vi "ReversedEngineering GetDiagramSubVIs.vi"(0 "Diagram":refnum<vi>, 1 "SubVIsOptions(NormalSubVis)":T1(ring), 2 "RecrsiveSearchInNormalSubVIs(False)":bool, 5 "error in (no error)":errorcluster, 9 "PathToDebugVI(OnlyUsedForRecursivVitFiles)":path) -> (14 "DiagramOut":refnum<vi>, 15 "SubViNames":string[](array[string]), 19 "error out":errorcluster)   [LabVIEW 2020]
panel:
  in  "Debug?":bool
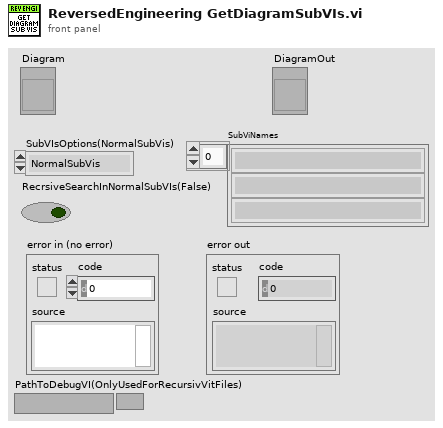
[diagram p1: front panel]
types:
  T1 = enum16{"NormalSubVis", "LV-Internal VIs", "All VIs", "All Functions"}
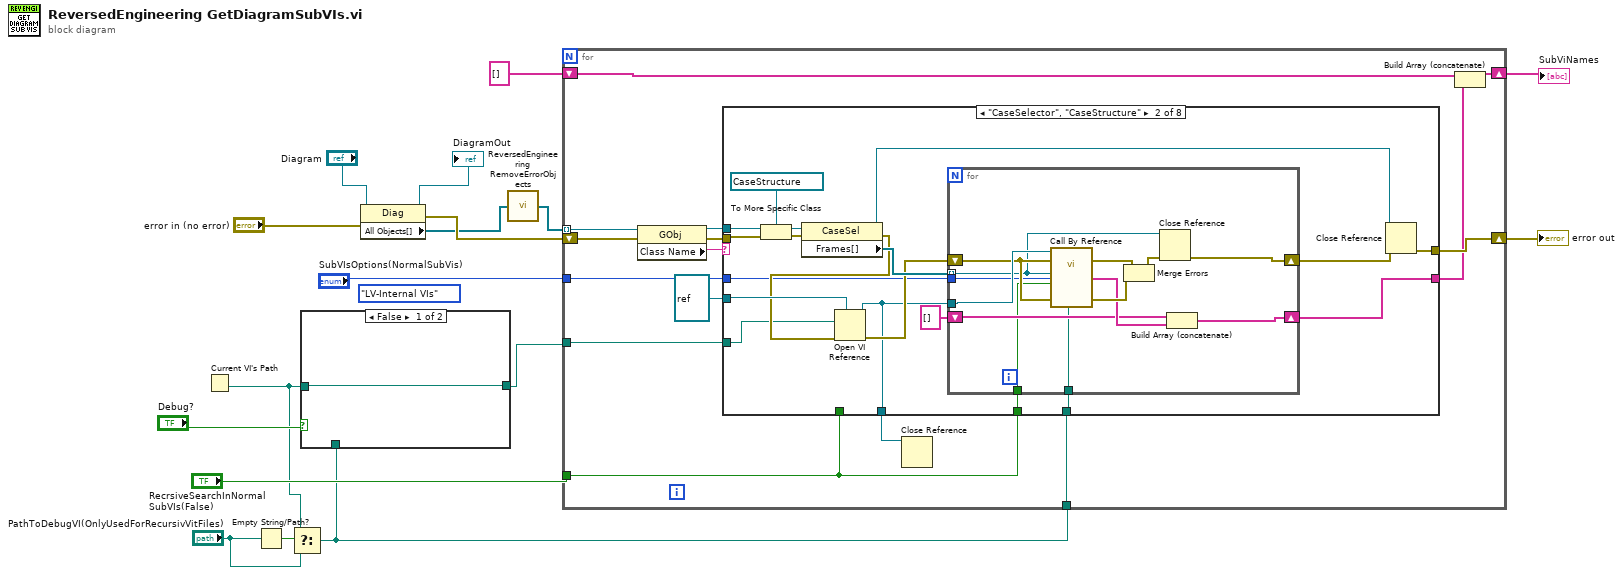
[diagram p0: block diagram]
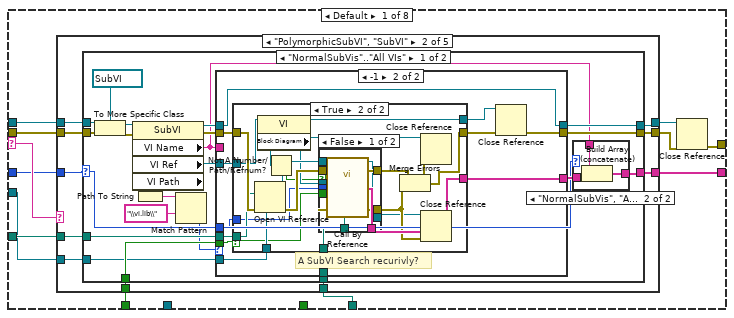
[diagram p2: hidden frame]
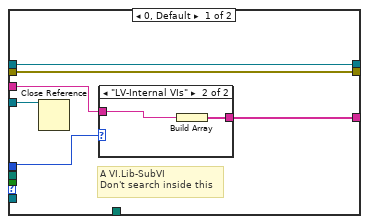
[diagram p5: hidden frame]
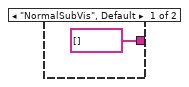
[diagram p6: hidden frame]
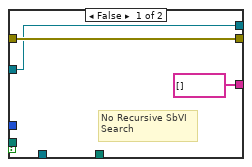
[diagram p7: hidden frame]
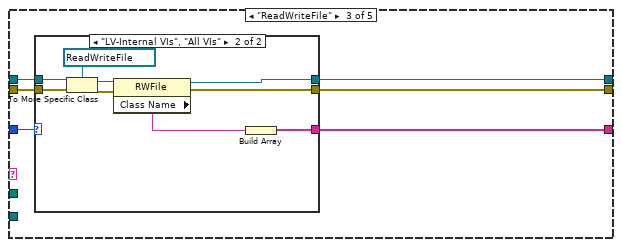
[diagram p10: hidden frame]
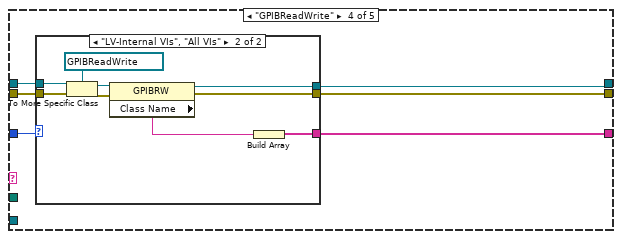
[diagram p12: hidden frame]
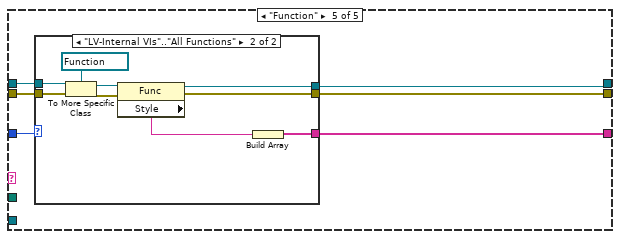
[diagram p14: hidden frame]
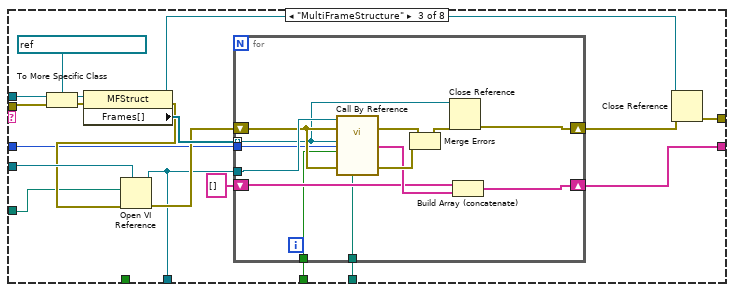
[diagram p16: hidden frame]
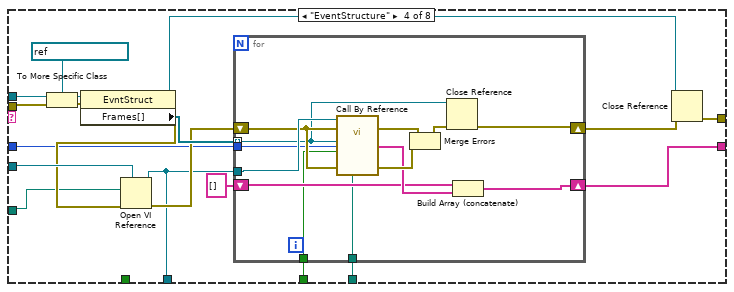
[diagram p17: hidden frame]
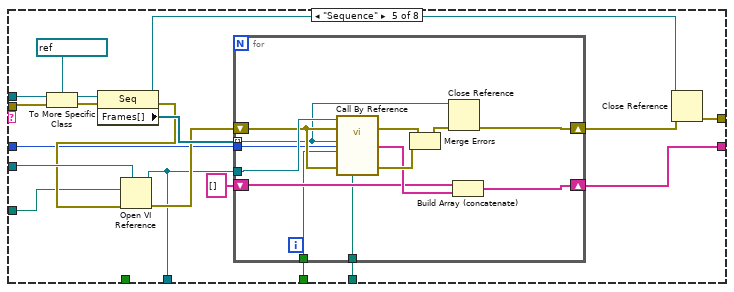
[diagram p18: hidden frame]
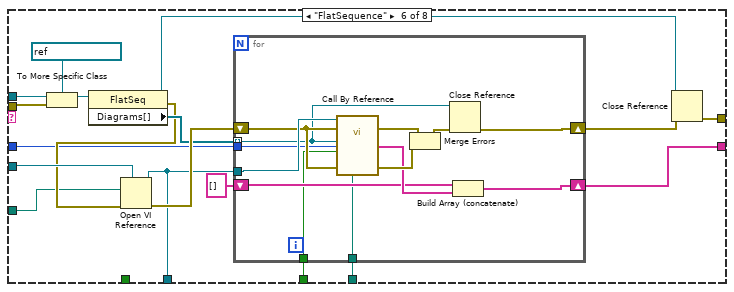
[diagram p19: hidden frame]
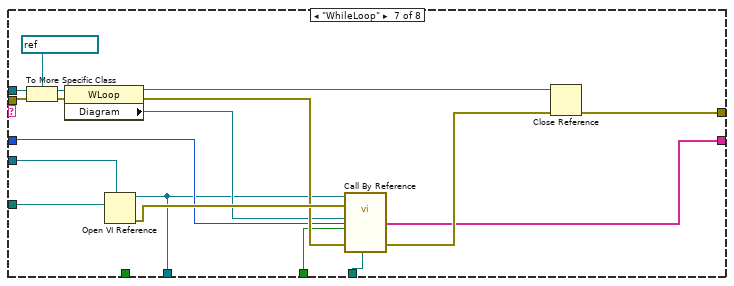
[diagram p20: hidden frame]
diagram:
  (unwired) T1."LV-Internal VIs" ("SubVIsOptions(NormalSubVis)")
  n1 = Current VI's Path() -> (path=w5:path)
  n2 = Empty String/Path?(string/path="PathToDebugVI(OnlyUsedForRecursivVitFiles)") -> (empty?=w6:bool)
  n3 = Select(t=w5, s=w6, f="PathToDebugVI(OnlyUsedForRecursivVitFiles)") -> (s? t:f=w3:path)
  n4 = case shown="False" "Debug?" {
    tunnel: w5 -> [w18 _]
    tunnel: [w18 w24] -> w8
    tunnel: w3 -> [_ w21]
    frame False {
    }
    frame True {
      n5 = Strip Path(path=w21) -> (stripped path=w19:path, name=w20:string)
      n6 = Concatenate Strings(w20, "t" ("f")) -> (w23:string)
      n7 = Build Path(base path=w19, name or relative path=w23) -> (appended path=w24:path)
    }
  }
  n8 = property class="Diag"(reference="Diagram", error in="error in (no error)") -> (reference out=→"DiagramOut":refnum<vi>, error out=w15:errorcluster, "All Objects[]"=w2:refnum<vi>[])
  n9 = call <resource>:"ReversedEngineering RemoveErrorObjects.vi"("ObjectsIn"=w2) -> ("ObjectsOut"=w1:refnum<vi>[])
  n10 = for {
    tunnel: w1 -> [w25] mode=indexing
    shift-right: [w38] -> w14
    shift-left: w15 -> [w39]
    shift-right: [w37] -> w13
    shift-left: string[] [] -> [w31]
    tunnel: w8 -> [w35]
    tunnel: "SubVIsOptions(NormalSubVis)" -> [w34]
    tunnel: "RecrsiveSearchInNormalSubVIs(False)" -> [w33]
    tunnel: w3 -> [w32]
    n11 = property class="GObj"(reference=w25, error in=w39) -> (reference out=w29:refnum<vi>, error out=w28:errorcluster, "Class Name"=w30:string)
    n12 = case shown="\"CaseSelector\", \"CaseStructure\"" w30 {
      selector: w30 -> [w50 _ _ _ _ _ _ _]
      tunnel: w29 -> [w48 w214 w246 w278 w310 w341 w372 w390]
      tunnel: w28 -> [w49 w209 w242 w274 w306 w340 w366 w384]
      tunnel: [w51 w208 w241 w273 w305 w339 w356 w374] -> w38
      tunnel: [w45 w202 w235 w267 w300 w335 w362 w380] -> w36
      tunnel: refnum<vi> refnum ("VI Refnum") -> [w41 w205 w238 w270 w302 w337 w361 w379]
      tunnel: w35 -> [w42 w200 w232 w264 w297 w328 w360 w378]
      tunnel: [_ w199 w231 w263 w295 w327 w355 w373] -> w26
      tunnel: w34 -> [w44 w198 w230 w262 w294 w326 w359 w377]
      tunnel: w33 -> [_ w197 w229 w261 w293 w325 w358 w376]
      tunnel: w33 -> [w43 _ _ _ _ _ _ _]
      tunnel: w32 -> [w40 w196 w228 w260 w292 w324 w357 w375]
      frame Default {
        n13 = case shown="\"PolymorphicSubVI\", \"SubVI\"" w50 {
          tunnel: w49 -> [w53 w62 w149 w166 w183]
          tunnel: w48 -> [w52 w63 w150 w167 w184]
          tunnel: [w53 w60 w147 w162 w179] -> w47
          tunnel: [w52 w59 w146 w164 w181] -> w46
          tunnel: [_ w61 w148 w165 w182] -> w45
          tunnel: w44 -> [_ w58 w145 w163 w180]
          tunnel: w43 -> [_ w57 _ _ _]
          tunnel: w42 -> [_ w56 _ _ _]
          tunnel: w41 -> [_ w55 _ _ _]
          tunnel: w40 -> [_ w54 _ _ _]
          frame "False", Default {
          }
          frame "PolymorphicSubVI", "SubVI" {
            n14 = case shown="\"NormalSubVis\"..\"All VIs\"" w58 {
              selector: w58 -> [w66 _]
              tunnel: w63 -> [w84 w144]
              tunnel: w62 -> [w83 w143]
              tunnel: [w81 _] -> w61
              tunnel: [w73 w143] -> w60
              tunnel: [w74 w144] -> w59
              tunnel: w57 -> [w71 _]
              tunnel: w56 -> [w70 _]
              tunnel: w55 -> [w68 _]
              tunnel: w54 -> [w67 _]
              frame "NormalSubVis".."All VIs" {
                n15 = To More Specific Class(target class=refnum<vi> refnum ("WhileLoop"), reference=w84, error in=w83) -> (specific class reference=w82:refnum<vi>, error out=w80:errorcluster)
                n16 = property class="SubVI"(reference=w82, error in=w80) -> (reference out=w75:refnum<vi>, error out=w76:errorcluster, "VI Name"=w64:string, "VI Ref"=w69:refnum<vi>, "VI Path"=w79:path)
                n17 = Path To String(path=w79) -> (string=w78:string)
                n18 = Match Pattern(string=w78, regular expression="\\vi.lib\\") -> (offset past match=w65:i32)  [unwired: 4 out]
                n19 = case shown="-1" w65 {
                  tunnel: w76 -> [w94 w109]
                  tunnel: w75 -> [w95 w102]
                  tunnel: [w95 w102] -> w74
                  tunnel: [w94 w100] -> w73
                  tunnel: [w92 w108] -> w72
                  tunnel: w71 -> [_ w110]
                  tunnel: w70 -> [_ w107]
                  tunnel: w69 -> [w93 w106]
                  tunnel: w68 -> [_ w105]
                  tunnel: w67 -> [_ w104]
                  tunnel: w66 -> [w91 w103]
                  tunnel: w64 -> [w90 _]
                  frame 0, Default {
                    # "A VI.Lib-SubVI\nDon't search inside this"
                    n20 = Close Reference(reference=w93) -> ()  [unwired: 1 in, 1 out]
                    n21 = case shown="\"LV-Internal VIs\"" w91 {
                      tunnel: [string[] [] w98] -> w92
                      tunnel: w90 -> [_ w97]
                      frame "NormalSubVis", Default {
                      }
                      frame "LV-Internal VIs" {
                        n22 = Build Array(w97) -> (w98:string[])
                      }
                    }
                  }
                  frame -1 {
                    # "A SubVI Search recurivly?"
                    n23 = case shown="True" w110 {
                      selector: w110 -> [_ w121]
                      tunnel: w109 -> [w113 w128]
                      tunnel: [w113 w115] -> w101
                      tunnel: [string[] [] ("appended array") w123] -> w108
                      tunnel: w107 -> [_ w127]
                      tunnel: w106 -> [w111 w125]
                      tunnel: w105 -> [_ w124]
                      tunnel: w103 -> [_ w122]
                      tunnel: w104 -> [_ w118]
                      tunnel: [w111 w114] -> w99
                      frame False {
                        # "No Recursive SbVI\nSearch"
                      }
                      frame True {
                        n24 = Open VI Reference(type specifier VI Refnum (for type only)=w124, vi path=w127, error in (no error)=w128) -> (vi reference=w126:refnum<vi>, error out=w129:errorcluster)  [unwired: 3 out]
                        n25 = property class="VI"(reference=w125) -> (reference out=w114:refnum<vi>, "Block Diagram"=w117:refnum<vi>)  [unwired: 1 in, 1 out]
                        n26 = Not A Number/Path/Refnum?(number/path/refnum=w117) -> (NaN/Path/Refnum?=w116:bool)
                        n27 = case shown="False" w116 {
                          tunnel: [w140 w142] -> w130
                          tunnel: w129 -> [w139 w142]
                          tunnel: w126 -> [w138 w141]
                          tunnel: w117 -> [w137 _]
                          tunnel: [w136 _] -> w123
                          tunnel: w122 -> [w135 _]
                          tunnel: w121 -> [w134 _]
                          tunnel: [w133 _] -> w120
                          tunnel: [w132 w141] -> w119
                          tunnel: w118 -> [w131 _]
                          frame False {
                            n28 = call-by-ref "?"(reference=w138, error in=w139, "Diagram"=w137, "SubVIsOptions(NormalSubVis)"=w135, "RecrsiveSearchInNormalSubVIs(False)"=w134, "error in (no error)"=w139, "PathToDebugVI(OnlyUsedForRecursivVitFiles)"=w131) -> (reference out=w132:refnum<vi>, error out=w140:errorcluster, "SubViNames"=w136:string[], 19:"error out"=w133:errorcluster)  [unwired: 12 in, 1 out]
                          }
                          frame True {
                          }
                        }
                        n29 = Merge Errors(w130, w120) -> (w115:errorcluster)
                        n30 = Close Reference(reference=w117, error in (no error)=w115) -> ()  [unwired: 1 out]
                        n31 = Close Reference(reference=w119, error in (no error)=w120) -> ()  [unwired: 1 out]
                      }
                    }
                    n32 = Close Reference(reference=w99, error in (no error)=w101) -> (error out=w100:errorcluster)
                  }
                }
                n33 = case shown="\"NormalSubVis\", \"All VIs\"" w66 {
                  tunnel: [w86 w89] -> w81
                  tunnel: w64 -> [_ w88]
                  tunnel: w72 -> [w86 w87]
                  frame Default {
                  }
                  frame "NormalSubVis", "All VIs" {
                    n34 = Build Array (concatenate)(w88, w87) -> (w89:string[])
                  }
                }
              }
              frame Default {
              }
            }
          }
          frame "ReadWriteFile" {
            n35 = case shown="\"LV-Internal VIs\", \"All VIs\"" w145 {
              tunnel: w150 -> [w152 w160]
              tunnel: w149 -> [w151 w159]
              tunnel: [_ w156] -> w148
              tunnel: [w151 w155] -> w147
              tunnel: [w152 w154] -> w146
              frame Default {
              }
              frame "LV-Internal VIs", "All VIs" {
                n36 = To More Specific Class(target class=refnum<vi> refnum ("WhileLoop"), reference=w160, error in=w159) -> (specific class reference=w158:refnum<vi>, error out=w153:errorcluster)
                n37 = property class="RWFile"(reference=w158, error in=w153) -> (reference out=w154:refnum<vi>, error out=w155:errorcluster, "Class Name"=w157:string)
                n38 = Build Array(w157) -> (w156:string[])
              }
            }
          }
          frame "GPIBReadWrite" {
            n39 = case shown="\"LV-Internal VIs\", \"All VIs\"" w163 {
              tunnel: w167 -> [w169 w177]
              tunnel: w166 -> [w168 w176]
              tunnel: [_ w173] -> w165
              tunnel: [w169 w172] -> w164
              tunnel: [w168 w170] -> w162
              frame Default {
              }
              frame "LV-Internal VIs", "All VIs" {
                n40 = To More Specific Class(target class=refnum<vi> refnum ("WhileLoop"), reference=w177, error in=w176) -> (specific class reference=w175:refnum<vi>, error out=w171:errorcluster)
                n41 = property class="GPIBRW"(reference=w175, error in=w171) -> (reference out=w172:refnum<vi>, error out=w170:errorcluster, "Class Name"=w174:string)
                n42 = Build Array(w174) -> (w173:string[])
              }
            }
          }
          frame "Function" {
            n43 = case shown="\"LV-Internal VIs\"..\"All Functions\"" w180 {
              tunnel: w184 -> [w186 w194]
              tunnel: w183 -> [w185 w193]
              tunnel: [_ w190] -> w182
              tunnel: [w186 w189] -> w181
              tunnel: [w185 w187] -> w179
              frame Default {
              }
              frame "LV-Internal VIs".."All Functions" {
                n44 = To More Specific Class(target class=refnum<vi> refnum ("WhileLoop"), reference=w194, error in=w193) -> (specific class reference=w192:refnum<vi>, error out=w188:errorcluster)
                n45 = property class="Func"(reference=w192, error in=w188) -> (reference out=w189:refnum<vi>, error out=w187:errorcluster, "Style"=w191:string)
                n46 = Build Array(w191) -> (w190:string[])
              }
            }
          }
        }
        n47 = Close Reference(reference=w46, error in (no error)=w47) -> (error out=w51:errorcluster)
      }
      frame "CaseSelector", "CaseStructure" {
        n48 = To More Specific Class(target class=refnum<vi> refnum ("CaseSelector"), reference=w214, error in=w209) -> (specific class reference=w212:refnum<vi>, error out=w210:errorcluster)
        n49 = property class="CaseSel"(reference=w212, error in=w210) -> (reference out=w206:refnum<vi>, error out=w204:errorcluster, "Frames[]"=w211:refnum<vi>[])
        n50 = Open VI Reference(type specifier VI Refnum (for type only)=w205, vi path=w200, error in (no error)=w204) -> (vi reference=w199:refnum<vi>, error out=w207:errorcluster)  [unwired: 3 out]
        n51 = for {
          tunnel: w211 -> [w218] mode=indexing
          shift-right: [w220] -> w203
          shift-left: w207 -> [w225]
          tunnel: w199 -> [w226]
          shift-right: [w221] -> w202
          shift-left: string[] [] -> [w222]
          tunnel: w198 -> [w217]
          tunnel: w197 -> [w216]
          tunnel: w196 -> [w215]
          n52 = call-by-ref "?"(reference=w226, error in=w225, "Diagram"=w218, "SubVIsOptions(NormalSubVis)"=w217, "RecrsiveSearchInNormalSubVIs(False)"=w216, "error in (no error)"=w225, "PathToDebugVI(OnlyUsedForRecursivVitFiles)"=w215) -> (error out=w227:errorcluster, "SubViNames"=w223:string[], 19:"error out"=w224:errorcluster)  [unwired: 12 in, 2 out]
          n53 = Merge Errors(w227, w224) -> (w219:errorcluster)
          n54 = Close Reference(reference=w218, error in (no error)=w219) -> (error out=w220:errorcluster)
          n55 = Build Array (concatenate)(w222, w223) -> (w221:string[])
        }
        n56 = Close Reference(reference=w206, error in (no error)=w203) -> (error out=w208:errorcluster)
      }
      frame "MultiFrameStructure" {
        n57 = To More Specific Class(target class=refnum<vi> refnum ("MultiFrameStructure"), reference=w246, error in=w242) -> (specific class reference=w245:refnum<vi>, error out=w243:errorcluster)
        n58 = property class="MFStruct"(reference=w245, error in=w243) -> (reference out=w239:refnum<vi>, error out=w237:errorcluster, "Frames[]"=w244:refnum<vi>[])
        n59 = Open VI Reference(type specifier VI Refnum (for type only)=w238, vi path=w232, error in (no error)=w237) -> (vi reference=w231:refnum<vi>, error out=w240:errorcluster)  [unwired: 3 out]
        n60 = for {
          tunnel: w244 -> [w252] mode=indexing
          shift-right: [w250] -> w236
          shift-left: w240 -> [w257]
          tunnel: w231 -> [w258]
          shift-right: [w253] -> w235
          shift-left: string[] [] -> [w254]
          tunnel: w230 -> [w249]
          tunnel: w229 -> [w248]
          tunnel: w228 -> [w247]
          n61 = call-by-ref "?"(reference=w258, error in=w257, "Diagram"=w252, "SubVIsOptions(NormalSubVis)"=w249, "RecrsiveSearchInNormalSubVIs(False)"=w248, "error in (no error)"=w257, "PathToDebugVI(OnlyUsedForRecursivVitFiles)"=w247) -> (error out=w259:errorcluster, "SubViNames"=w255:string[], 19:"error out"=w256:errorcluster)  [unwired: 12 in, 2 out]
          n62 = Merge Errors(w259, w256) -> (w251:errorcluster)
          n63 = Close Reference(reference=w252, error in (no error)=w251) -> (error out=w250:errorcluster)
          n64 = Build Array (concatenate)(w254, w255) -> (w253:string[])
        }
        n65 = Close Reference(reference=w239, error in (no error)=w236) -> (error out=w241:errorcluster)
      }
      frame "EventStructure" {
        n66 = To More Specific Class(target class=refnum<vi> refnum ("EventStructure"), reference=w278, error in=w274) -> (specific class reference=w277:refnum<vi>, error out=w275:errorcluster)
        n67 = property class="EvntStruct"(reference=w277, error in=w275) -> (reference out=w271:refnum<vi>, error out=w269:errorcluster, "Frames[]"=w276:refnum<vi>[])
        n68 = Open VI Reference(type specifier VI Refnum (for type only)=w270, vi path=w264, error in (no error)=w269) -> (vi reference=w263:refnum<vi>, error out=w272:errorcluster)  [unwired: 3 out]
        n69 = for {
          tunnel: w276 -> [w282] mode=indexing
          shift-right: [w283] -> w268
          shift-left: w272 -> [w289]
          tunnel: w263 -> [w290]
          shift-right: [w285] -> w267
          shift-left: string[] [] -> [w286]
          tunnel: w262 -> [w281]
          tunnel: w261 -> [w280]
          tunnel: w260 -> [w279]
          n70 = call-by-ref "?"(reference=w290, error in=w289, "Diagram"=w282, "SubVIsOptions(NormalSubVis)"=w281, "RecrsiveSearchInNormalSubVIs(False)"=w280, "error in (no error)"=w289, "PathToDebugVI(OnlyUsedForRecursivVitFiles)"=w279) -> (error out=w291:errorcluster, "SubViNames"=w287:string[], 19:"error out"=w288:errorcluster)  [unwired: 12 in, 2 out]
          n71 = Merge Errors(w291, w288) -> (w284:errorcluster)
          n72 = Close Reference(reference=w282, error in (no error)=w284) -> (error out=w283:errorcluster)
          n73 = Build Array (concatenate)(w286, w287) -> (w285:string[])
        }
        n74 = Close Reference(reference=w271, error in (no error)=w268) -> (error out=w273:errorcluster)
      }
      frame "Sequence" {
        n75 = To More Specific Class(target class=refnum<vi> refnum ("Sequence"), reference=w310, error in=w306) -> (specific class reference=w309:refnum<vi>, error out=w307:errorcluster)
        n76 = property class="Seq"(reference=w309, error in=w307) -> (reference out=w303:refnum<vi>, error out=w301:errorcluster, "Frames[]"=w308:refnum<vi>[])
        n77 = Open VI Reference(type specifier VI Refnum (for type only)=w302, vi path=w297, error in (no error)=w301) -> (vi reference=w295:refnum<vi>, error out=w304:errorcluster)  [unwired: 3 out]
        n78 = for {
          tunnel: w308 -> [w314] mode=indexing
          shift-right: [w316] -> w296
          shift-left: w304 -> [w321]
          tunnel: w295 -> [w322]
          shift-right: [w317] -> w300
          shift-left: string[] [] -> [w318]
          tunnel: w294 -> [w313]
          tunnel: w293 -> [w312]
          tunnel: w292 -> [w311]
          n79 = call-by-ref "?"(reference=w322, error in=w321, "Diagram"=w314, "SubVIsOptions(NormalSubVis)"=w313, "RecrsiveSearchInNormalSubVIs(False)"=w312, "error in (no error)"=w321, "PathToDebugVI(OnlyUsedForRecursivVitFiles)"=w311) -> (error out=w323:errorcluster, "SubViNames"=w319:string[], 19:"error out"=w320:errorcluster)  [unwired: 12 in, 2 out]
          n80 = Merge Errors(w323, w320) -> (w315:errorcluster)
          n81 = Close Reference(reference=w314, error in (no error)=w315) -> (error out=w316:errorcluster)
          n82 = Build Array (concatenate)(w318, w319) -> (w317:string[])
        }
        n83 = Close Reference(reference=w303, error in (no error)=w296) -> (error out=w305:errorcluster)
      }
      frame "FlatSequence" {
        n84 = To More Specific Class(target class=refnum<vi> refnum ("FlatSequence"), reference=w341, error in=w340) -> (specific class reference=w332:refnum<vi>)  [unwired: 1 out]
        n85 = property class="FlatSeq"(reference=w332) -> (reference out=w329:refnum<vi>, error out=w330:errorcluster, "Diagrams[]"=w331:refnum<vi>[])  [unwired: 1 in]
        n86 = Open VI Reference(type specifier VI Refnum (for type only)=w337, vi path=w328, error in (no error)=w330) -> (vi reference=w327:refnum<vi>, error out=w338:errorcluster)  [unwired: 3 out]
        n87 = for {
          tunnel: w331 -> [w345] mode=indexing
          shift-right: [w347] -> w336
          shift-left: w338 -> [w352]
          tunnel: w327 -> [w353]
          shift-right: [w348] -> w335
          shift-left: string[] [] -> [w349]
          tunnel: w326 -> [w344]
          tunnel: w325 -> [w343]
          tunnel: w324 -> [w342]
          n88 = call-by-ref "?"(reference=w353, error in=w352, "Diagram"=w345, "SubVIsOptions(NormalSubVis)"=w344, "RecrsiveSearchInNormalSubVIs(False)"=w343, "error in (no error)"=w352, "PathToDebugVI(OnlyUsedForRecursivVitFiles)"=w342) -> (error out=w354:errorcluster, "SubViNames"=w350:string[], 19:"error out"=w351:errorcluster)  [unwired: 12 in, 2 out]
          n89 = Merge Errors(w354, w351) -> (w346:errorcluster)
          n90 = Close Reference(reference=w345, error in (no error)=w346) -> (error out=w347:errorcluster)
          n91 = Build Array (concatenate)(w349, w350) -> (w348:string[])
        }
        n92 = Close Reference(reference=w329, error in (no error)=w336) -> (error out=w339:errorcluster)
      }
      frame "WhileLoop" {
        n93 = To More Specific Class(target class=refnum<vi> refnum ("WhileLoop"), reference=w372, error in=w366) -> (specific class reference=w371:refnum<vi>, error out=w367:errorcluster)
        n94 = property class="WLoop"(reference=w371, error in=w367) -> (reference out=w369:refnum<vi>, error out=w364:errorcluster, "Diagram"=w363:refnum<vi>)
        n95 = Open VI Reference(type specifier VI Refnum (for type only)=w361, vi path=w360) -> (vi reference=w355:refnum<vi>, error out=w368:errorcluster)  [unwired: 1 in, 3 out]
        n96 = call-by-ref "?"(reference=w355, error in=w368, "Diagram"=w363, "SubVIsOptions(NormalSubVis)"=w359, "RecrsiveSearchInNormalSubVIs(False)"=w358, "error in (no error)"=w364, "PathToDebugVI(OnlyUsedForRecursivVitFiles)"=w357) -> ("SubViNames"=w362:string[], "error out"=w365:errorcluster)  [unwired: 12 in, 3 out]
        n97 = Close Reference(reference=w369, error in (no error)=w365) -> (error out=w356:errorcluster)
      }
      frame "ForLoop" {
        n98 = To More Specific Class(target class=refnum<vi> refnum ("WhileLoop"), reference=w390, error in=w384) -> (specific class reference=w389:refnum<vi>, error out=w385:errorcluster)
        n99 = property class="FLoop"(reference=w389, error in=w385) -> (reference out=w387:refnum<vi>, error out=w382:errorcluster, "Diagram"=w381:refnum<vi>)
        n100 = Open VI Reference(type specifier VI Refnum (for type only)=w379, vi path=w378) -> (vi reference=w373:refnum<vi>, error out=w386:errorcluster)  [unwired: 1 in, 3 out]
        n101 = call-by-ref "?"(reference=w373, error in=w386, "Diagram"=w381, "SubVIsOptions(NormalSubVis)"=w377, "RecrsiveSearchInNormalSubVIs(False)"=w376, "error in (no error)"=w382, "PathToDebugVI(OnlyUsedForRecursivVitFiles)"=w375) -> ("SubViNames"=w380:string[], "error out"=w383:errorcluster)  [unwired: 12 in, 3 out]
        n102 = Close Reference(reference=w387, error in (no error)=w383) -> (error out=w374:errorcluster)
      }
    }
    n103 = Close Reference(reference=w26) -> ()  [unwired: 1 in, 1 out]
    n104 = Build Array (concatenate)(w31, w36) -> (w37:string[])
  }
  "error out" <- w14
  "SubViNames" <- w13
